vi "Init VMR.vi"(8 "error in (no error)":errorcluster, 11 "VMR Actor in":refnum<class "VMR Actor.lvclass">) -> (0 "error out":errorcluster, 3 "VMR Actor out":refnum<class "VMR Actor.lvclass">)   [LabVIEW 2022 SP3, in "VMR Server.lvlib" / "VMR Actor.lvclass"]
uses:
  VMR Actor.lvclass
  VMR Actor.lvclass/VMR Actor.ctl
  <vilib>/IlluminatedG/IG VoicemeeterRemote API/VoiceMeeterRemote/VoiceMeeterRemote/VoiceMeeterRemote.lvclass
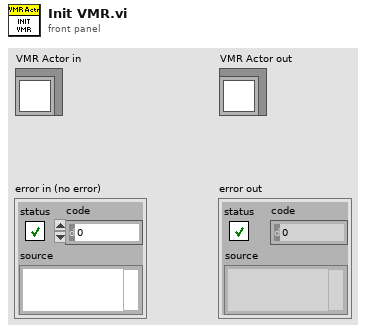
[diagram p1: front panel]
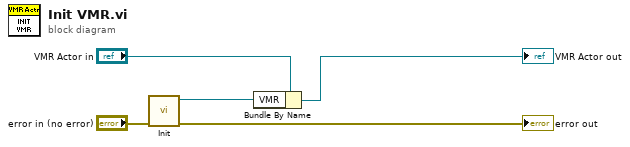
[diagram p0: block diagram]
diagram:
  n1 = call <vilib>:"Init.vi"("error in (no error)"="error in (no error)") -> ("error out"=→"error out":errorcluster, "VoiceMeeterRemote out"=w5:refnum<class "VoiceMeeterRemote.lvclass">)  [unwired: 8 in, 1 out]
  n2 = Bundle By Name(cluster="VMR Actor in", "VMR"=w5) -> (→"VMR Actor out":refnum<class "VMR Actor.lvclass">)
